vi "Util_Progress Show Progress Popup.vi"(8 "error in (no error)":errorcluster, 9 "Title":string, 10 "Message":string) -> (0 "error out":errorcluster)   [LabVIEW 2016]
panel:
  out "appended path":path
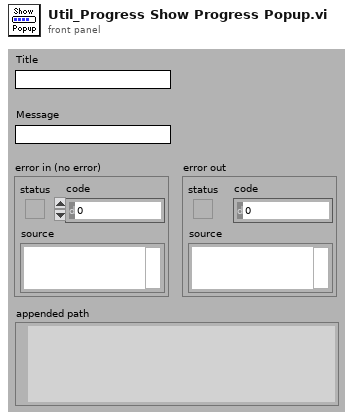
[diagram p1: front panel]
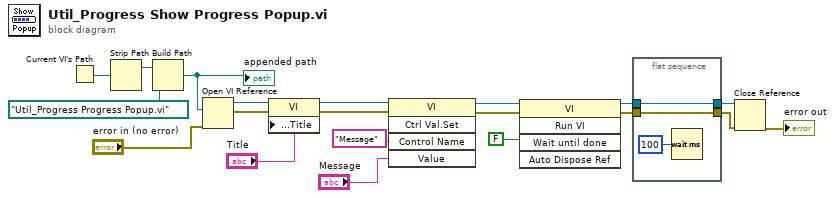
[diagram p0: block diagram]
diagram:
  n1 = Current VI's Path() -> (path=w10:path)
  n2 = Strip Path(path=w10) -> (stripped path=w9:path)  [unwired: 1 out]
  n3 = Build Path(base path=w9, name or relative path=path "Util_Progress Progress Popup.vi" ("vi path")) -> (appended path=w7:path)
  "appended path" <- w7
  n4 = Open VI Reference(vi path=w7, error in (no error)="error in (no error)") -> (vi reference=w19:refnum<vi>, error out=w20:errorcluster)  [unwired: 4 out]
  n5 = property class="VI"(reference=w19, error in=w20, "Front Panel.Title"="Title") -> (reference out=w14:refnum<vi>, error out=w15:errorcluster)
  n6 = invoke class="VI" method="Ctrl Val.Set"(reference=w14, error in=w15, "Control Name"="Message", "Value"="Message") -> (reference out=w1:refnum<vi>, error out=w2:errorcluster)  [unwired: 1 in, 3 out]
  n7 = invoke class="VI" method="Run VI"(reference=w1, error in=w2, "Wait until done"=FALSE ("Wait Until Done")) -> (reference out=w6:refnum<vi>, error out=w4:errorcluster)  [unwired: 2 in, 3 out]
  n8 = flat-sequence {
    tunnel: [w23] -> w5
    tunnel: w6 -> [w23]
    tunnel: [w22] -> w3
    tunnel: w4 -> [w22]
    frame #0 {
      n9 = Wait (ms)(milliseconds to wait=u32 100) -> ()  [unwired: 1 out]
    }
  }
  n10 = Close Reference(reference=w5, error in (no error)=w3) -> (error out=→"error out":errorcluster)
